vi "lvSetConditionalSymbol.vi"() -> (0 "error out":errorcluster)   [LabVIEW 2014, in "lvcommonbuild.lvlib"]
uses:
  lvcommonbuild.lvlib
  <vilib>/Wiresmith Technology/LabVIEW CLI/CLI Class/CLI.lvclass
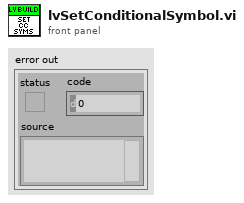
[diagram p1: front panel]
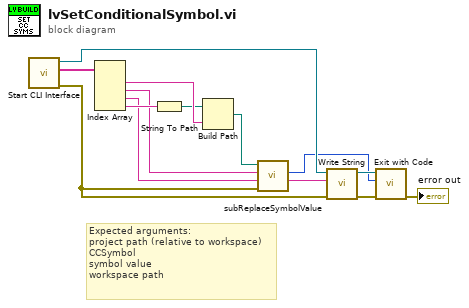
[diagram p0: block diagram]
diagram:
  # "Expected arguments:\nproject path (relative to workspace)\nCCSymbol\nsymbol value\nworkspace path"
  n1 = call <vilib>:"Start CLI Interface.vi"() -> ("error out"=w7:errorcluster, "Custom Parameters"=w14:string[], "CLI out"=w12:refnum<class "CLI.lvclass">)  [unwired: 9 in]
  n2 = Index Array(array=w14) -> (element #1=w6:string, element #2=w1:string, element #3=w2:string, element #4=w5:string)  [unwired: 4 in]
  n3 = String To Path(string=w5) -> (path=w4:path)
  n4 = Build Path(base path=w4, name or relative path=w6) -> (appended path=w3:path)
  n5 = call "subReplaceSymbolValue.vi"("error in (no error)"=w7, "Value"=w2, "Symbol"=w1, "Project Path"=w3) -> ("Output Message"=w13:string, "Exit Code"=w9:i32)  [unwired: 5 in, 1 out]
  n6 = call <vilib>:"Write String.vi"("error in (no error)"=w7, "Text to Write"=w13, "CLI in"=w12) -> ("error out"=w11:errorcluster, "CLI out"=w10:refnum<class "CLI.lvclass">)  [unwired: 7 in]
  n7 = call <vilib>:"Exit with Code.vi"("error in (no error)"=w11, "Exit Code (0)"=w9, "CLI in"=w10) -> ("error out"=→"error out":errorcluster)  [unwired: 8 in]
